vi "Handle Drag Starting.vi"(4 "Mods":cluster{"Double Click":bool, "Menu Key":bool}, 5 "Drag Mode":enum32{"copy or move", "copy only", "move only"}(ring), 6 "PlatMods":T3, 7 "Button":u16, 8 "error in (no error)":errorcluster, 9 "Coords":T2, 10 "Data":T4(array[cluster]), 11 "File Explorer in":refnum<class "File Explorer.lvclass">) -> (0 "error out":errorcluster, 2 "Drag Starting Filtered Event Data":T1, 3 "File Explorer out":refnum<class "File Explorer.lvclass">)   [LabVIEW 2020, in "File Explorer.lvlib" / "File Explorer.lvclass"]
uses:
  <vilib>/gpm_packages/@cs/file-explorer-extension/Source/File Explorer/File Explorer/File Explorer.lvclass
  <vilib>/Utility/miscctls.llb/LVPoint32TypeDef.ctl
  <vilib>/gpm_packages/@cs/file-explorer-extension/Source/Application Dependencies/Application Types/Drag Starting Filtered Event Data.ctl
  <vilib>/gpm_packages/@cs/file-explorer-extension/Source/File Explorer/File Explorer.lvlib
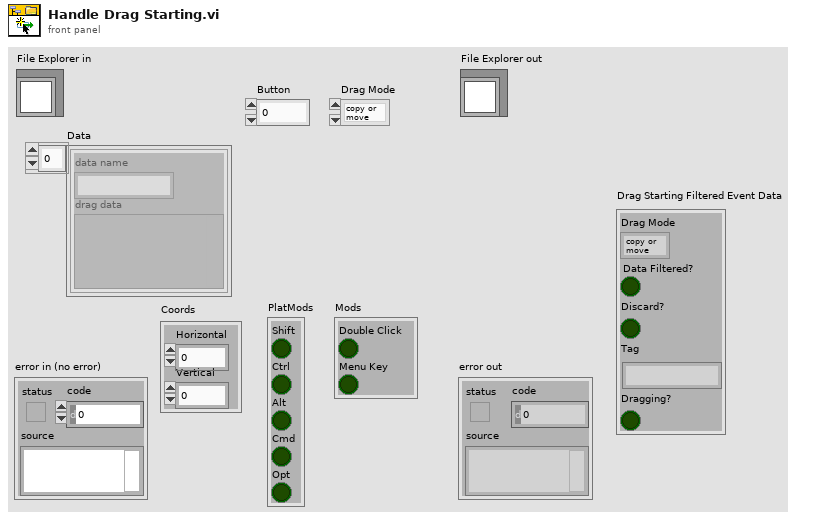
[diagram p1: front panel]
types:
  T1 = typedef "File Explorer.lvlib/Drag Starting Filtered Event Data.ctl" = cluster{"Drag Mode":enum32{"copy or move", "copy only", "move only"}, "Data Filtered?":bool, "Discard?":bool, "Tag":string, "Dragging?":bool}
  T2 = typedef "LVPoint32TypeDef.ctl" = cluster{"Horizontal":i32, "Vertical":i32}
  T3 = cluster{"Shift":bool, "Ctrl":bool, "Alt":bool, "Cmd":bool, "Opt":bool}
  T4 = cluster{"data name":string, "drag data":variant}[]
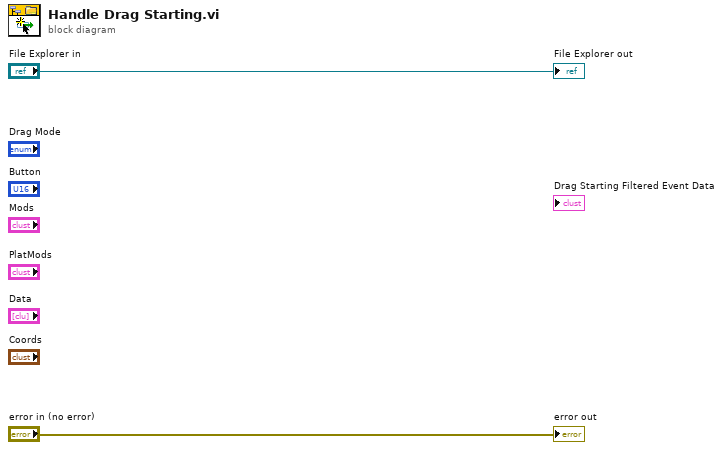
[diagram p0: block diagram]
diagram:
  "error out" <- "error in (no error)"
  "File Explorer out" <- "File Explorer in"
